vi "Heater Status.vi"(8 "error in (no error)":errorcluster, 10 "Loop (1:Loop 1)":u16(ring)=1 items=["Loop 1"=1, "Loop 2"=2], 11 "VISA resource name":refnum<visa-resource-name>) -> (0 "error out":errorcluster, 1 "Heater Range":enum16{"Off", "Low", "High"}(ring), 3 "VISA resource name out":refnum<visa-resource-name>)   [LabVIEW 2019, in "Lake Shore 325.lvlib"]
uses:
  Lake Shore 325.lvlib
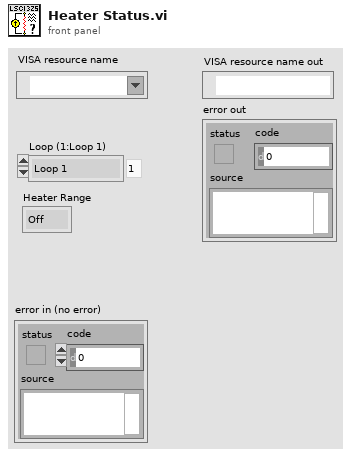
[diagram p1: front panel]
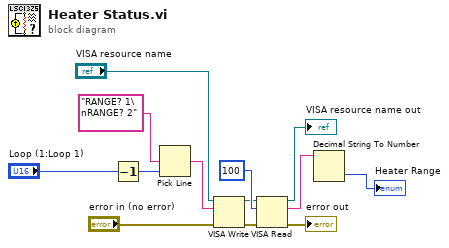
[diagram p0: block diagram]
diagram:
  n1 = Decrement(x="Loop (1:Loop 1)") -> (x-1=w9:u16)
  n2 = Pick Line(multi-line string="RANGE? 1\nRANGE? 2", line index=w9) -> (output string=w5:string)  [unwired: 1 in]
  n3 = VISA Write(VISA resource name="VISA resource name", write buffer=w5, error in (no error)="error in (no error)") -> (VISA resource name out=w7:refnum<visa-resource-name>, error out=w6:errorcluster)  [unwired: 1 out]
  n4 = VISA Read(VISA resource name=w7, byte count=100, error in (no error)=w6) -> (VISA resource name out=→"VISA resource name out":refnum<visa-resource-name>, read buffer=w2:string, error out=→"error out":errorcluster)  [unwired: 1 out]
  n5 = Decimal String To Number(string=w2) -> (number=→"Heater Range":i32)  [unwired: 2 in, 1 out]
